vi "Frameremap.vi"(11 "Frame Parameters (m)":T1) -> (0 "FH (nm)":dbl, 1 "FW (nm)":dbl, 2 "Z Origin (nm)":dbl, 3 "X Origin (nm)":dbl)   [LabVIEW 2019]
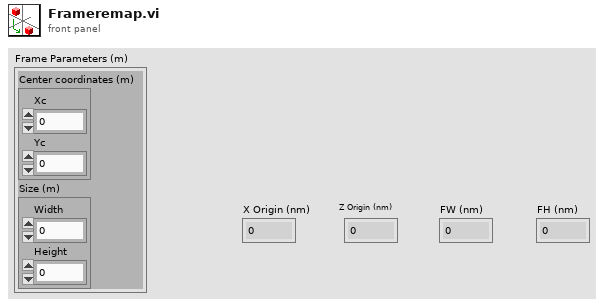
[diagram p1: front panel]
types:
  T1 = cluster{"Center coordinates (m)":cluster{"Xc":sgl, "Yc":sgl}, "Size (m)":cluster{"Width":sgl, "Height":sgl}}
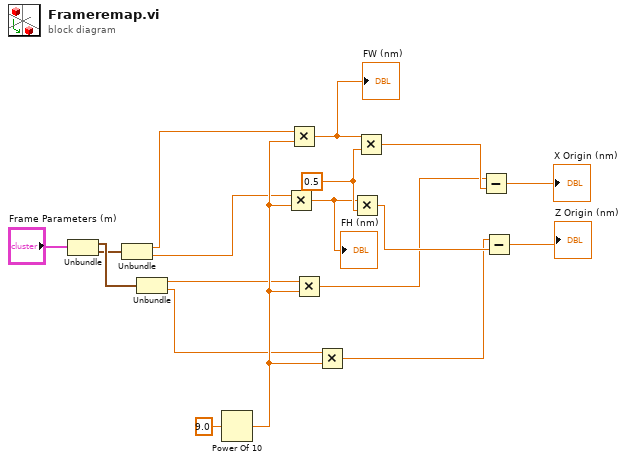
[diagram p0: block diagram]
diagram:
  w18 = 0.5 ("y")
  n1 = Unbundle("Frame Parameters (m)") -> ("Center coordinates (m)"=w6:cluster{"Xc":sgl, "Yc":sgl}, "Size (m)"=w3:cluster{"Width":sgl, "Height":sgl})
  n2 = Unbundle(w3) -> ("Width"=w2:sgl, "Height"=w1:sgl)
  n3 = Unbundle(w6) -> ("Xc"=w5:sgl, "Yc"=w4:sgl)
  n4 = Power Of 10(x=9.0) -> (10^x=w8:dbl)
  n5 = Multiply(x=w1, y=w8) -> (x*y=w12:dbl)
  "FH (nm)" <- w12
  n6 = Multiply(x=w2, y=w8) -> (x*y=w13:dbl)
  "FW (nm)" <- w13
  n7 = Multiply(x=w5, y=w8) -> (x*y=w11:dbl)
  n8 = Multiply(x=w4, y=w8) -> (x*y=w10:dbl)
  n9 = Multiply(x=w12, y=w18) -> (x*y=w16:dbl)
  n10 = Multiply(x=w13, y=w18) -> (x*y=w17:dbl)
  n11 = Subtract(x=w11, y=w17) -> (x-y=→"X Origin (nm)":dbl)
  n12 = Subtract(x=w10, y=w16) -> (x-y=→"Z Origin (nm)":dbl)
